vi "Write IMAQ Image.vi"(0 "image in":refnum<class "MSC Image.lvclass">, 5 "error in (no error)":errorcluster) -> (14 "image out":refnum<class "MSC Image.lvclass">, 15 "IMAQ Image out":T1, 19 "error out":errorcluster)   [LabVIEW 2014, in "MSC Image.lvclass"]
doc: "Converts a MSC Image to an IMAQ Image. \n\nThe IMAQ image occupies memory. Use IMAQ Dispose to clear it when you dont need it anymore."
uses:
  MSC Image.lvclass
  <vilib>/vision/Image Controls.llb/IMAQ Image.ctl
  MSC Image.lvclass/MSC Image.ctl
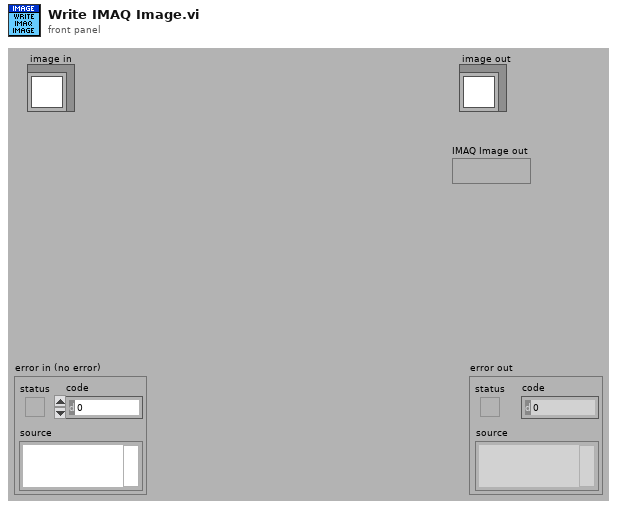
[diagram p1: front panel]
types:
  T1 = typedef "IMAQ Image.ctl" = refnum<image>
  T2 = typedef "MSC Image.lvclass/Image Type.ctl" = i32
  T3 = typedef "Image Type" = u32
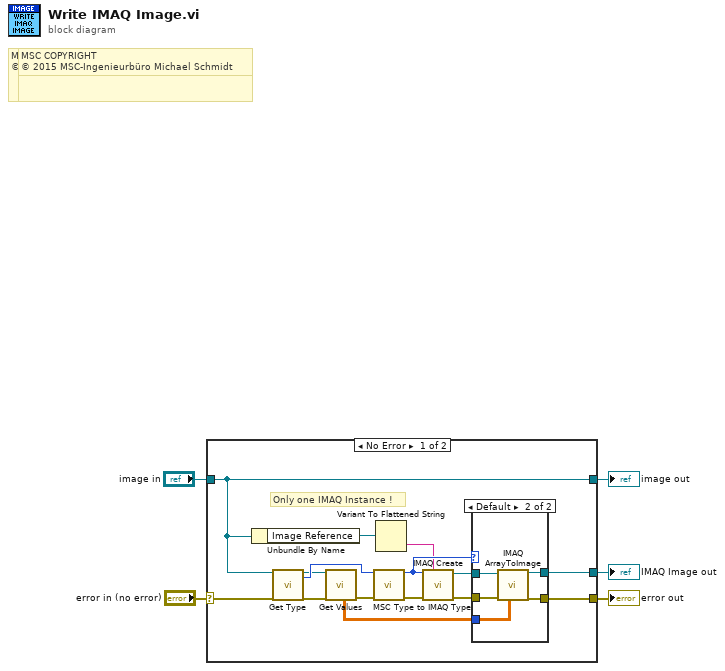
[diagram p0: block diagram]
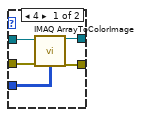
[diagram p2: hidden frame]
diagram:
  # "MSC COPYRIGHT\n© 2016 MSC-Ingenieurbüro Michael Schmidt"
  # "MSC COPYRIGHT\n© 2016 MSC-Ingenieurbüro Michael Schmidt"
  # "MSC COPYRIGHT\n© 2015 MSC-Ingenieurbüro Michael Schmidt"
  # "MSC COPYRIGHT\n© 2015 MSC-Ingenieurbüro Michael Schmidt"
  n1 = case shown="No Error" "error in (no error)" {
    selector: "error in (no error)" -> [w8 w37]
    tunnel: [w7 w37] -> w4
    tunnel: [w6 w36] -> w2
    tunnel: "image in" -> [w6 w36]
    tunnel: [w9 _] -> w1
    frame No Error {
      # "Only one IMAQ Instance !"
      n2 = Unbundle By Name(w6) -> ("Image Reference"=w19:refnum<data-value>)
      n3 = call-dynamic "Get Type.vi"("image in"=w6, "error in (no error)"=w8) -> ("image out"=w17:refnum<class "MSC Image.lvclass">, "Image Type"=w18:T2, "error out"=w16:errorcluster)  [unwired: 15 in]
      n4 = call-dynamic "Get Values.vi"("image in"=w17, "error in (no error)"=w16) -> ("imageData BGR"=w12:u32[][], "imageData U8"=w11:u8[][], "imageData U16"=w10:u16[][], "imageData Single"=w14:sgl[][], "error out"=w15:errorcluster)  [unwired: 10 in, 3 out]
      n5 = call "MSC Type to IMAQ Type.vi"("MSC Picture Type"=w18, "error in (no error)"=w15) -> ("IMAQ Type"=w23:T3, "error out"=w22:errorcluster)  [unwired: 12 in]
      n6 = Variant To Flattened String(Variant=w19) -> (data string=w13:string)  [unwired: 1 out]
      n7 = call "IMAQ Create"("Image Name"=w13, "Image Type"=w23, "error in (no error)"=w22) -> ("New Image"=w21:T1, "error out"=w20:errorcluster)  [unwired: 2 in]
      n8 = case shown="Default" w23 {
        tunnel: w20 -> [w27 w35]
        tunnel: w21 -> [w28 w34]
        tunnel: w14 -> [_ w33]
        tunnel: [w26 w32] -> w7
        tunnel: [w25 w31] -> w9
        tunnel: w12 -> [w24 _]
        tunnel: w11 -> [_ w30]
        tunnel: w10 -> [_ w29]
        frame 4 {
          n9 = call "IMAQ ArrayToColorImage"("Image Pixels (U32)"=w24, "Image"=w28, "error in (no error)"=w27) -> ("Image Out"=w25:T1, "error out"=w26:errorcluster)  [unwired: 2 in]
        }
        frame Default {
          n10 = call "IMAQ ArrayToImage"("Image Pixels (Float)"=w33, "Image Pixels (U16)"=w29, "error in (no error)"=w35, "Image Pixels (U8)"=w30, "Image"=w34) -> ("error out"=w32:errorcluster, "Image Out"=w31:T1)  [unwired: 5 in]
        }
      }
    }
    frame Error {
    }
  }
  "error out" <- w4
  "image out" <- w2
  "IMAQ Image out" <- w1
